vi "Hormiga_Close.vi"(1 "error in (no error)":errorcluster, 3 "VISA Refnum in":refnum<visa-resource-name>) -> ()   [LabVIEW 2016]
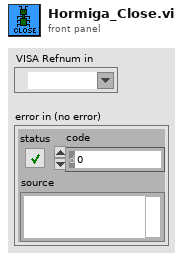
[diagram p1: front panel]
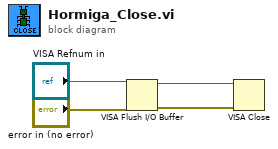
[diagram p0: block diagram]
diagram:
  n1 = VISA Flush I/O Buffer(VISA resource name="VISA Refnum in", error in (no error)="error in (no error)") -> (VISA resource name out=w3:refnum<visa-resource-name>, error out=w2:errorcluster)  [unwired: 1 in]
  n2 = VISA Close(VISA resource name=w3, error in (no error)=w2) -> ()  [unwired: 1 out]
